vi "EQE_main_Ver2.vi"() -> ()   [LabVIEW 2017]
uses:
  <vilib>/Utility/file.llb/Write Delimited Spreadsheet (DBL).vi
  Documents/Data/Chunxiong Bao/Capacitance/SR830/Stanford Research 830/Stanford Research 830.lvlib
  Program Files (x86)/Bentham/SDK/code examples/LabView/8.0/BenHw/benhw32_stdcall.dll
panel:
  out "System Setup 2":i32
  out "Park":i32
  in  "Calibration":bool
  in  "Close Program":bool
  in  "Scan":bool
  in  "Tab Control":T1(tab)
  in  "Calibration detector":enum16{"Silicon", "Germanium", "InGaAs"}(ring)
  in  "Save path":path
  in  "Device name":string
  in  "Start Wl":dbl=300.0
  in  "Stop Wl":dbl=1000.0
  in  "Step":dbl=5.0
  in  "CFG File":path=path "C:/Users/Biorgel/Desktop/EQE/Configuration Files/system.cfg"
  in  "ATR File":path=path "C:/Users/Biorgel/Desktop/EQE/Configuration Files/system.atr"
  in  "VISA LOCK-IN":refnum<visa-resource-name>="GPIB0::8::INSTR"
  in  "Input Connection (0: Single-Ended Voltage)":u16(ring) items=["Single-Ended Voltage", "Differential Voltage", "1 MOhm Current Gain", "100 MOhm Current Gain"]
  in  "Input Coupling (0: AC)":u16(ring) items=["AC", "DC"]
  in  "Dynamic Reserve (2: Low Noise)":i8(ring) items=["High Reserve"=0, "Normal"=1, "Low Noise"=2, "Auto Reserve"=-1]
  in  "Sensitivity (26: 1 V/uA)":i8(ring)=26 items=["Auto Gain"=-1, "2 nV/fA"=0, "5 nV/fA"=1, "10 nV/fA"=2, "20 nV/fA"=3, "50 nV/fA"=4, "100 nV/fA"=5, "200 nV/fA"=6, "500 nV/fA"=7, "1 uV/pA"=8, "2 uV/pA"=9, "5 uV/pA"=10, "10 uV/pA"=11, "20 uV/pA"=12, "50 uV/pA"=13, "100 uV/pA"=14, "200 uV/pA"=15, "500 uV/pA"=16, "1 mV/nA"=17, "2 mV/nA"=18, "5 mV/nA"=19, "10 mV/nA"=20, "20 mV/nA"=21, "50 mV/nA"=22, "100 mV/nA"=23, "200 mV/nA"=24, "500 mV/mA"=25, "1 V/uA"=26]
  in  "Sine Output Amplitude (1 V)":dbl=1.0
  in  "Internal Reference Frequency (1000 Hz)":dbl=1000.0
  in  "Input Shield Grounding (0: Float)":u16(ring)=1 items=["Float", "Ground"]
  in  "Time Constant (8: 100ms)":u16(ring)=8 items=["10 us", "30 us", "100 us", "300 us", "1 ms", "3 ms", "10 ms", "30 ms", "100 ms", "300 ms", "1 s", "3 s", "10 s", "30 s", "100 s", "300 s", "1 ks", "3 ks", "10 ks", "30 ks"]
  in  "Start Park":bool
  in  "Move to Wavelength":bool
  out "Scan Error Code":i32
  out "System Setup":i32
  out "Current Wavelength":dbl
  out "Error Code":i32
  in  "Input Wavelength":dbl
  out "EQE graph":cluster{dbl[], dbl[]}(graph)
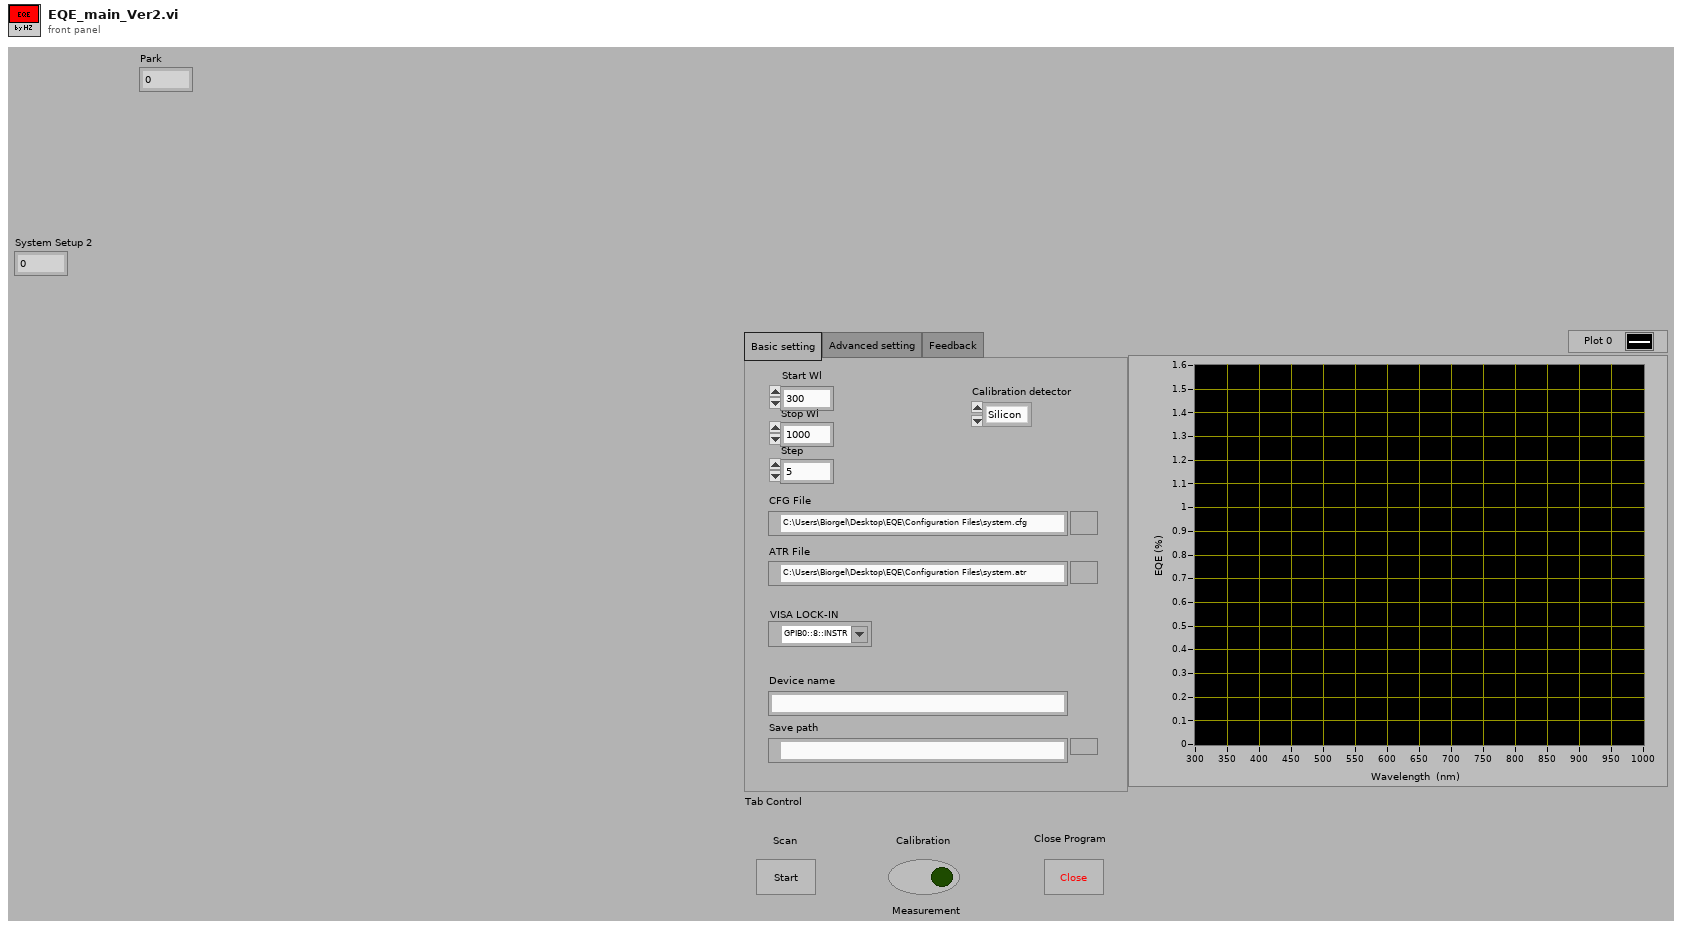
[diagram p1: front panel]
types:
  T1 = enum32{"Basic setting", "Advanced setting", "Feedback"}
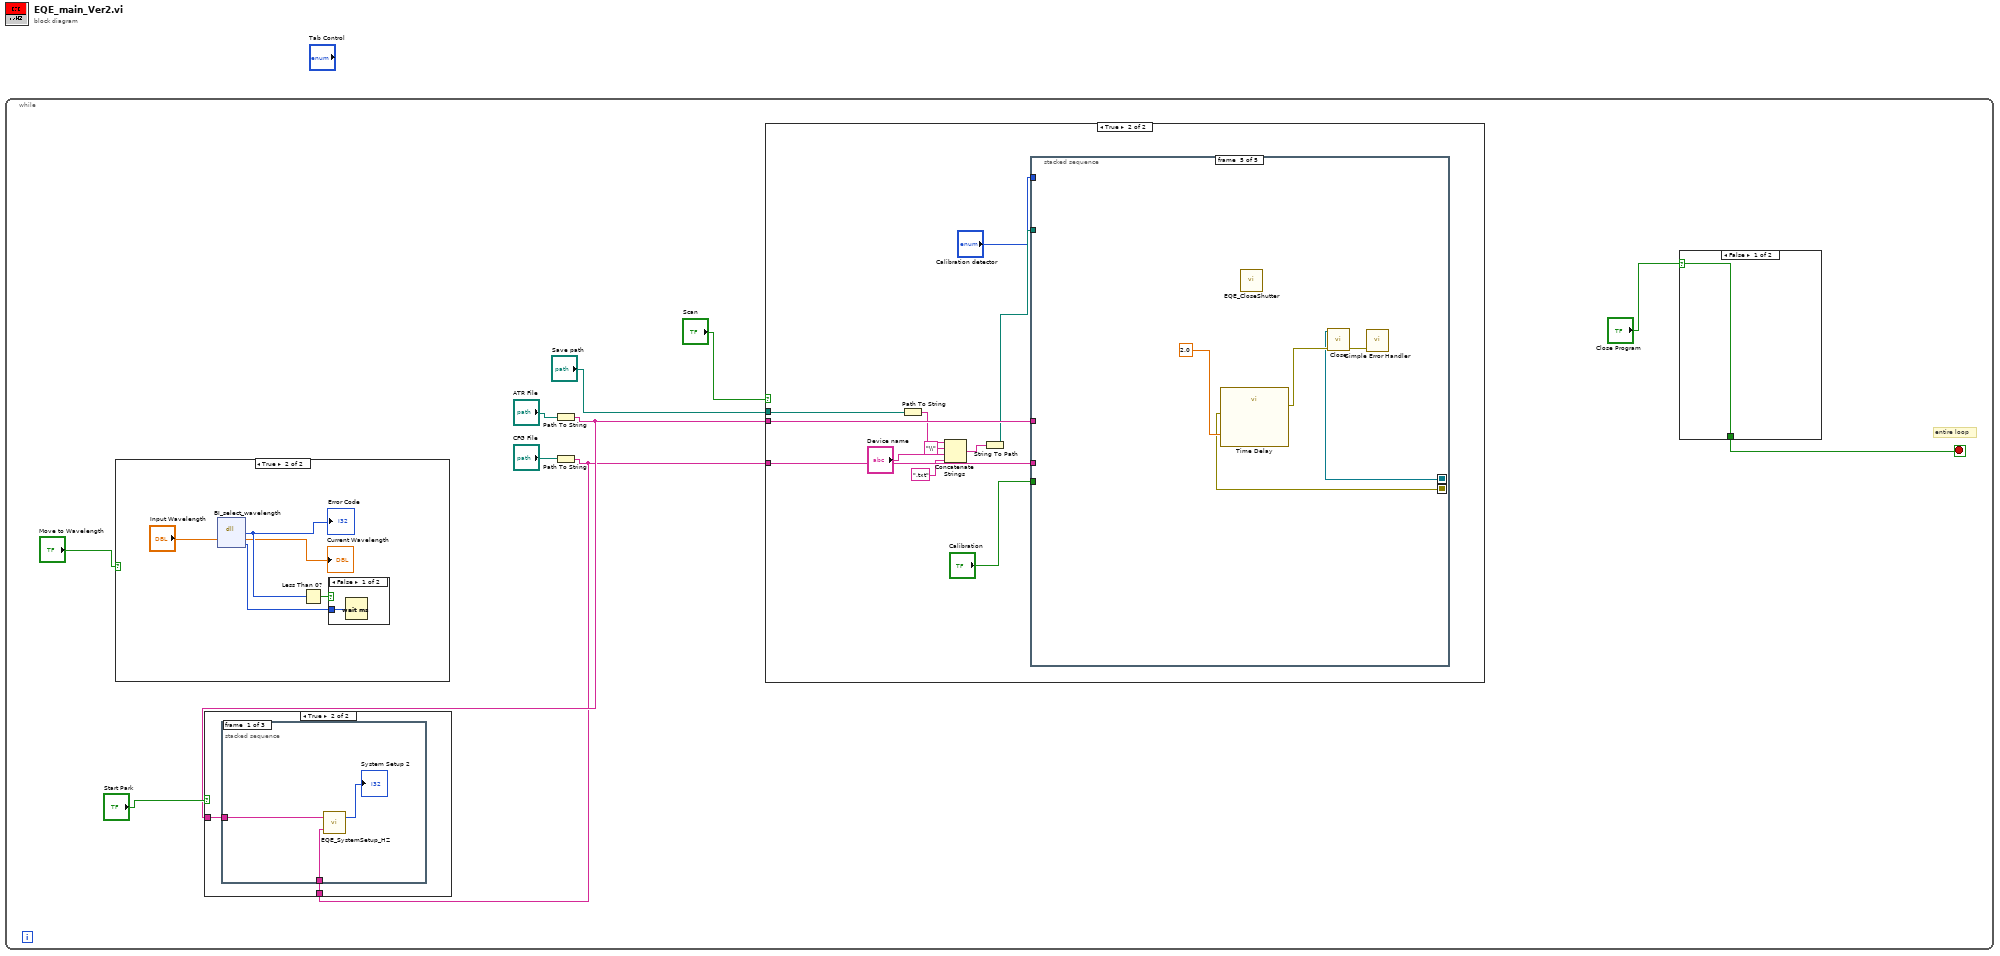
[diagram p0: block diagram]
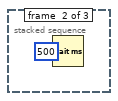
[diagram p3: hidden frame]
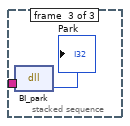
[diagram p4: hidden frame]
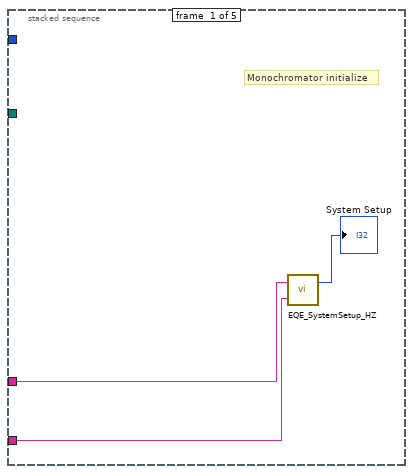
[diagram p8: hidden frame]
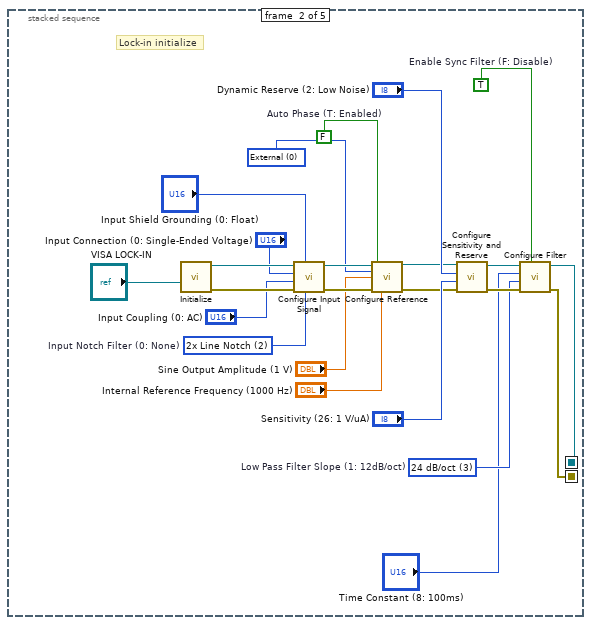
[diagram p9: hidden frame]
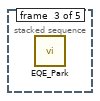
[diagram p10: hidden frame]
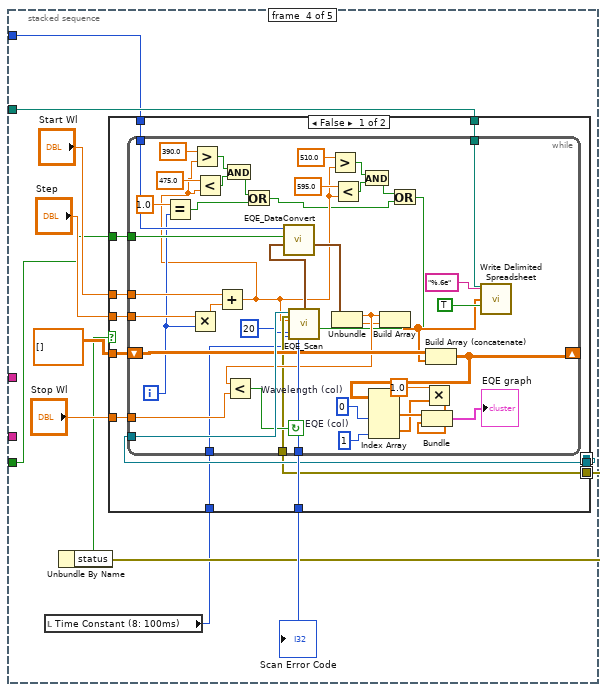
[diagram p11: hidden frame]
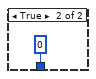
[diagram p12: hidden frame]
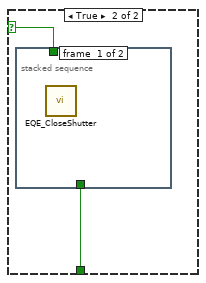
[diagram p13: hidden frame]
diagram:
  n1 = while {
    stop <- w9 stop-if-true
    # "entire loop"
    n2 = case shown="True" "Move to Wavelength" {
      frame False {
      }
      frame True {
        n3 = dll-call lib="C:/Program Files (x86)/Bentham/SDK/code examples/LabView/8.0/BenHw/benhw32_stdcall.dll" fn="BI_select_wavelength"("wl"="Input Wavelength") -> ("return type"=w22:i16, "wl"=→"Current Wavelength":dbl, "settle_delay"=w21:i32)  [unwired: 4 in, 2 out]
        "Error Code" <- w22
        n4 = Less Than 0?(x=w22) -> (x < 0?=w20:bool)
        n5 = case shown="False" w20 {
          tunnel: w21 -> [w23 _]
          frame False {
            n6 = Wait (ms)(milliseconds to wait=w23) -> ()  [unwired: 1 out]
          }
          frame True {
          }
        }
      }
    }
    n7 = Path To String(path="ATR File") -> (string=w2:string)
    n8 = Path To String(path="CFG File") -> (string=w1:string)
    n9 = case shown="True" "Start Park" {
      tunnel: w1 -> [_ w12]
      tunnel: w2 -> [_ w11]
      frame False {
      }
      frame True {
        n10 = stacked-sequence {
          tunnel: w11 -> [w14 _ _]
          tunnel: w12 -> [w13 _ _]
          frame #0 {
            n11 = call "EQE_SystemSetup_HZ.vi"("CFG File Path"=w13, "ATR File Path"=w14) -> ("Error Code"=→"System Setup 2":i32)  [unwired: 1 out]
          }
          frame #1 {
            n12 = Wait (ms)(milliseconds to wait=u32 500) -> ()  [unwired: 1 out]
          }
          frame #2 {
            n13 = dll-call lib="C:/Program Files (x86)/Bentham/SDK/code examples/LabView/8.0/BenHw/benhw32_stdcall.dll" fn="BI_park"() -> (→"Park":i16)  [unwired: 3 in, 2 out]
          }
        }
      }
    }
    n14 = case shown="True" "Scan" {
      tunnel: w1 -> [_ w34]
      tunnel: w2 -> [_ w33]
      tunnel: "Save path" -> [_ w24]
      frame False {
      }
      frame True {
        n15 = Path To String(path=w24) -> (string=w30:string)
        n16 = Concatenate Strings(w30, "\\" ("string"), "Device name", ".txt" ("string")) -> (w31:string)
        n17 = String To Path(string=w31) -> (path=w32:path)
        n18 = stacked-sequence {
          seq-local: [_ w40 _ _ _] -> [_ _ _ w66 w133]
          seq-local: [_ w39 _ _ _] -> [_ _ _ w70 w131]
          tunnel: w32 -> [_ _ _ w67 _]
          tunnel: "Calibration" -> [_ _ _ w64 _]
          tunnel: "Calibration detector" -> [_ _ _ w63 _]
          tunnel: w34 -> [w36 _ _ _ _]
          tunnel: w33 -> [w35 _ _ _ _]
          frame #0 {
            # "Monochromator initialize"
            n19 = call "EQE_SystemSetup_HZ.vi"("CFG File Path"=w36, "ATR File Path"=w35) -> ("Error Code"=→"System Setup":i32)  [unwired: 1 out]
          }
          frame #1 {
            w48 = u16 0 items=["External", "Internal"] ("Reference Source (1: Internal)")
            w42 = u16 3 items=["6 dB/oct", "12 dB/oct", "18 db/oct", "24 dB/oct"]  # Low Pass Filter Slope (1: 12dB/oct)
            w43 = TRUE  # Enable Sync Filter (F: Disable)
            w53 = FALSE  # Auto Phase (T: Enabled)
            w54 = u16 2 items=["None", "Line Notch", "2x Line Notch", "Both Notch Filters"]  # Input Notch Filter (0: None)
            # "Lock-in initialize"
            n20 = call "Initialize.vi"("VISA resource name"="VISA LOCK-IN") -> ("error out"=w61:errorcluster, "VISA resource name out"=w60:refnum<visa-resource-name>)  [unwired: 9 in]
            n21 = call "Configure Input Signal.vi"("Input Notch Filter (0: None)"=w54, "Input Shield Grounding (0: Float)"="Input Shield Grounding (0: Float)", "error in (no error)"=w61, "Input Coupling (0: AC)"="Input Coupling (0: AC)", "Input Connection (0: Single-Ended Voltage)"="Input Connection (0: Single-Ended Voltage)", "VISA resource name"=w60) -> ("error out"=w58:errorcluster, "VISA resource name out"=w59:refnum<visa-resource-name>)  [unwired: 4 in]
            n22 = call "Configure Reference.vi"("VISA resource name"=w59, "Auto Phase (T: Enabled)"=w53, "Reference Source (1: Internal)"=w48, "Sine Output Amplitude (1 V)"="Sine Output Amplitude (1 V)", "error in (no error)"=w58, "Internal Reference Frequency (1000 Hz)"="Internal Reference Frequency (1000 Hz)") -> ("VISA resource name out"=w50:refnum<visa-resource-name>, "error out"=w49:errorcluster)  [unwired: 8 in]
            n23 = call "Configure Sensitivity and Reserve.vi"("error in (no error)"=w49, "Sensitivity (-1: Auto gain)"="Sensitivity (26: 1 V/uA)", "Dynamic Reserve (-1: Auto Reserve)"="Dynamic Reserve (2: Low Noise)", "VISA resource name"=w50) -> ("error out"=w45:errorcluster, "VISA resource name out"=w44:refnum<visa-resource-name>)  [unwired: 6 in]
            n24 = call "Configure Filter.vi"("Enable Sync Filter (F: Disable)"=w43, "error in (no error)"=w45, "Low Pass Filter Slope (1: 12dB/oct)"=w42, "Time Constant (8: 100ms)"="Time Constant (8: 100ms)", "VISA resource name"=w44) -> ("error out"=w40:errorcluster, "VISA resource name out"=w39:refnum<visa-resource-name>)  [unwired: 5 in]
          }
          frame #2 {
            n25 = call "EQE_Park.vi"() -> ()  [unwired: 1 out]
          }
          frame #3 {
            n26 = local read "Time Constant (8: 100ms)"() -> (w62:u16)
            n27 = Unbundle By Name(w66) -> ("status"=w65:bool)
            n28 = case shown="False" w65 {
              tunnel: [w84 0 ("Error Code")] -> w73
              tunnel: "Start Wl" -> [w83 _]
              tunnel: "Step" -> [w82 _]
              tunnel: w70 -> [w81 _]
              tunnel: "Stop Wl" -> [w80 _]
              tunnel: dbl[][] [] -> [w79 _]
              tunnel: w67 -> [w78 _]
              tunnel: w66 -> [w77 _]
              tunnel: w64 -> [w76 _]
              tunnel: w63 -> [w75 _]
              tunnel: w62 -> [w74 _]
              frame False {
                n29 = while {
                  tunnel: [w129] -> w84
                  tunnel: w83 -> [w127]
                  tunnel: w82 -> [w126]
                  tunnel: w81 -> [w125]
                  tunnel: w80 -> [w124]
                  shift-right: [w115] -> _
                  shift-left: w79 -> [w122]
                  tunnel: w78 -> [w111]
                  tunnel: w77 -> [w110]
                  tunnel: w76 -> [w107]
                  tunnel: w75 -> [w106]
                  tunnel: w74 -> [w85]
                  i -> [w96]
                  stop <- w123 continue-if-true
                  w112 = 1  # EQE (col)
                  w113 = 0  # Wavelength (col)
                  n30 = Equal?(x=1.0, y=w96) -> (x = y?=w94:bool)
                  n31 = Multiply(x=w126, y=w96) -> (x*y=w128:dbl)
                  n32 = Add(x=w127, y=w128) -> (x+y=w89:dbl)
                  n33 = Greater?(x=390.0, y=w89) -> (0:w99:bool)
                  n34 = Less?(x=475.0, y=w89) -> (x < y?=w98:bool)
                  n35 = And(x=w99, y=w98) -> (x .and. y?=w95:bool)
                  n36 = Or(x=w95, y=w94) -> (x .or. y?=w87:bool)
                  n37 = Greater?(x=510.0, y=w89) -> (0:w91:bool)
                  n38 = Less?(x=595.0, y=w89) -> (x < y?=w90:bool)
                  n39 = And(x=w91, y=w90) -> (x .and. y?=w88:bool)
                  n40 = Or(x=w88, y=w87) -> (x .or. y?=w86:bool)
                  n41 = call "EQE_Scan.vi"("Max loop"=20, "error in (no error)"=w110, "milliseconds to wait"=w85, "Long delay"=w86, "Wavelength"=w89, "VISA Lock-in"=w125) -> ("Error Code"=w129:i32, "Output bundle"=w109:cluster{"Wavelength":dbl, "R":dbl})  [unwired: 1 in, 1 out]
                  n42 = call "EQE_DataConvert.vi"("Input"=w109, "Calibration"=w107, "Detector"=w106) -> ("Output"=w108:cluster{"Wavelength":dbl, "EQE":dbl})  [unwired: 8 in]
                  n43 = Unbundle(w108) -> ("Wavelength"=w121:dbl, "EQE"=w120:dbl)
                  n44 = Less?(x=w121, y=w124) -> (x < y?=w123:bool)
                  n45 = Build Array(w121, w120) -> (w117:dbl[])
                  n46 = Build Array (concatenate)(w122, w117) -> (w115:dbl[][])
                  n47 = Index Array(array=w115, index (col) #1=w113, index (col) #2=w112) -> (element #1=w114:dbl[], element #2=w105:dbl[])  [unwired: 2 in]
                  n48 = Multiply(x=1.0, y=w105) -> (x*y=w104:dbl[])
                  n49 = Bundle(w114, w104) -> (→"EQE graph":cluster{dbl[], dbl[]})  [unwired: 1 in]
                  n50 = call-poly <vilib>:"Write Delimited Spreadsheet.vi"("file path (dialog if empty)"=w111, "format (%.3f)"="%.6e", "1D data"=w117, "append to file? (new file:F)"=TRUE) -> ()  [unwired: 10 in, 2 out]
                }
              }
              frame True {
              }
            }
            "Scan Error Code" <- w73
          }
          frame #4 {
            n51 = call "Time Delay"("error in (no error)"=w133, "Delay Time (s)"=2.0) -> ("error out"=w132:errorcluster)  [unwired: 9 in]
            n52 = call "EQE_CloseShutter.vi"() -> ()  [unwired: 1 out]
            n53 = call "Close.vi"("error in (no error)"=w132, "VISA resource name"=w131) -> ("error out"=w134:errorcluster)  [unwired: 9 in]
            n54 = call <vilib>:"Simple Error Handler.vi"("error in (no error)"=w134) -> ()  [unwired: 4 in, 5 out]
          }
        }
      }
    }
    n55 = case shown="False" "Close Program" {
      selector: "Close Program" -> [w136 w138]
      tunnel: [w136 w137] -> w9
      frame False {
      }
      frame True {
        n56 = stacked-sequence {
          tunnel: w138 -> [_ w139]
          tunnel: [_ w139] -> w137
          frame #0 {
            n57 = call "EQE_CloseShutter.vi"() -> ()  [unwired: 1 out]
          }
          frame #1 {
          }
        }
      }
    }
  }
